vi "Characterise_Wind_Turbine.vi"(3 "Mode":T5, 5 "Traverse line In":T2 {"Row Duration (mins)" format="%#.1f"; "Row No" min=0; "Trace Gas Concentration (%)" min=0.0 format="%#.2f"; "Emission Rate (l/min)" format="%#.2f"; "Tunnel Speed" format="%#.2f"; "Start X" format="%#.2f"; "Start Y" format="%#.2f"; "Start Z" format="%#.2f"; "End X" format="%#.2f"; "End Y" format="%#.2f"; "End Z" format="%#.2f"; "Averaging time (min)" min=0.0 format="%#.2f"}) -> (0 "Error Message":string, 1 "Status":T1, 2 "Traverse line Out":T2 {"Row Duration (mins)" format="%#.1f"; "Row No" min=0; "Trace Gas Concentration (%)" min=0.0 format="%#.2f"; "Emission Rate (l/min)" format="%#.2f"; "Tunnel Speed" format="%#.2f"; "Start X" format="%#.2f"; "Start Y" format="%#.2f"; "Start Z" format="%#.2f"; "End X" format="%#.2f"; "End Y" format="%#.2f"; "End Z" format="%#.2f"; "Averaging time (min)" min=0.0 format="%#.2f"})   [LabVIEW 2010]
uses:
  Gen Trav/Multi_Run_Status.ctl
  Controls/Setup.ctl
  Controls/Save_Data.ctl
  Controls/Multi_run_mode.ctl
  Globals/Dynamic_call_global.ph.vi
  Plug in sub vis/Wind_Turbine_Global.vi
  Gen Trav/Spacing.ctl
  Gen Trav/Traverse_cluster.ctl
  Controls/User_Specific_mode.ctl
panel:
  out "Pitch Angle":dbl[](array[numeric])
  out "Array":dbl[][](array[numeric])=[[-2.5881, -0.8281, -0.8562, 5.2815, 2.845, -1.379, 0.12021, 0.04326, 0.05193, 200.0], [-3.9833, -4.1835, -3.2343, 3.6306, 1.4693, -1.9578, 0.016658, 0.014167, 0.012653, 150.0], [-9.3308, -8.7557, -8.688, 1.5839, 0.006762, -2.6254, 0.0025976, 0.0022319, 0.0025067, 100.0], [-22.4841, -21.7472, -21.4345, -1.4303, -2.2285, -3.8983, 0.00052601, 0.0020817, 0.00057503, 50.0], [-3.3014, -1.5466, -2.0325, 3.0316, -0.5057, -4.4498, 0.012392, 0.015677, 0.010797, 199.9955999515989], [-1.9125, -0.6788, -1.0112, 1.3489, -2.6429, -6.5215, 0.06848, 0.03886, 0.06433, 200.0]]
  out "Y=-200 X":dbl[](array[numeric])
  out "Y=200 X":dbl[](array[numeric])
  out "X below Highest point":dbl[](array[numeric])
  out "Yaw Angles":dbl[](array[numeric])
  out "Blade Angle":cluster{dbl[], dbl[]}[](graph)
  out "Index No":i32
  out "Current Case":string
  # "0 Blade 1 Angle\n1 Blade 2 Angle\n2 Blade 3 Angle\n3 Blade 1 Av X\n4 Blade 2 Av X\n5 Blade 3 Av X\n6 Blade 1 Var X\n7 Blade 2 Var X\n8 Blade 3 Var X\n9 Radius"
  # "X           Y            Z"
  # "Start"
  # "End"
  # "X           Y            Z"
  # "Start"
  # "End"
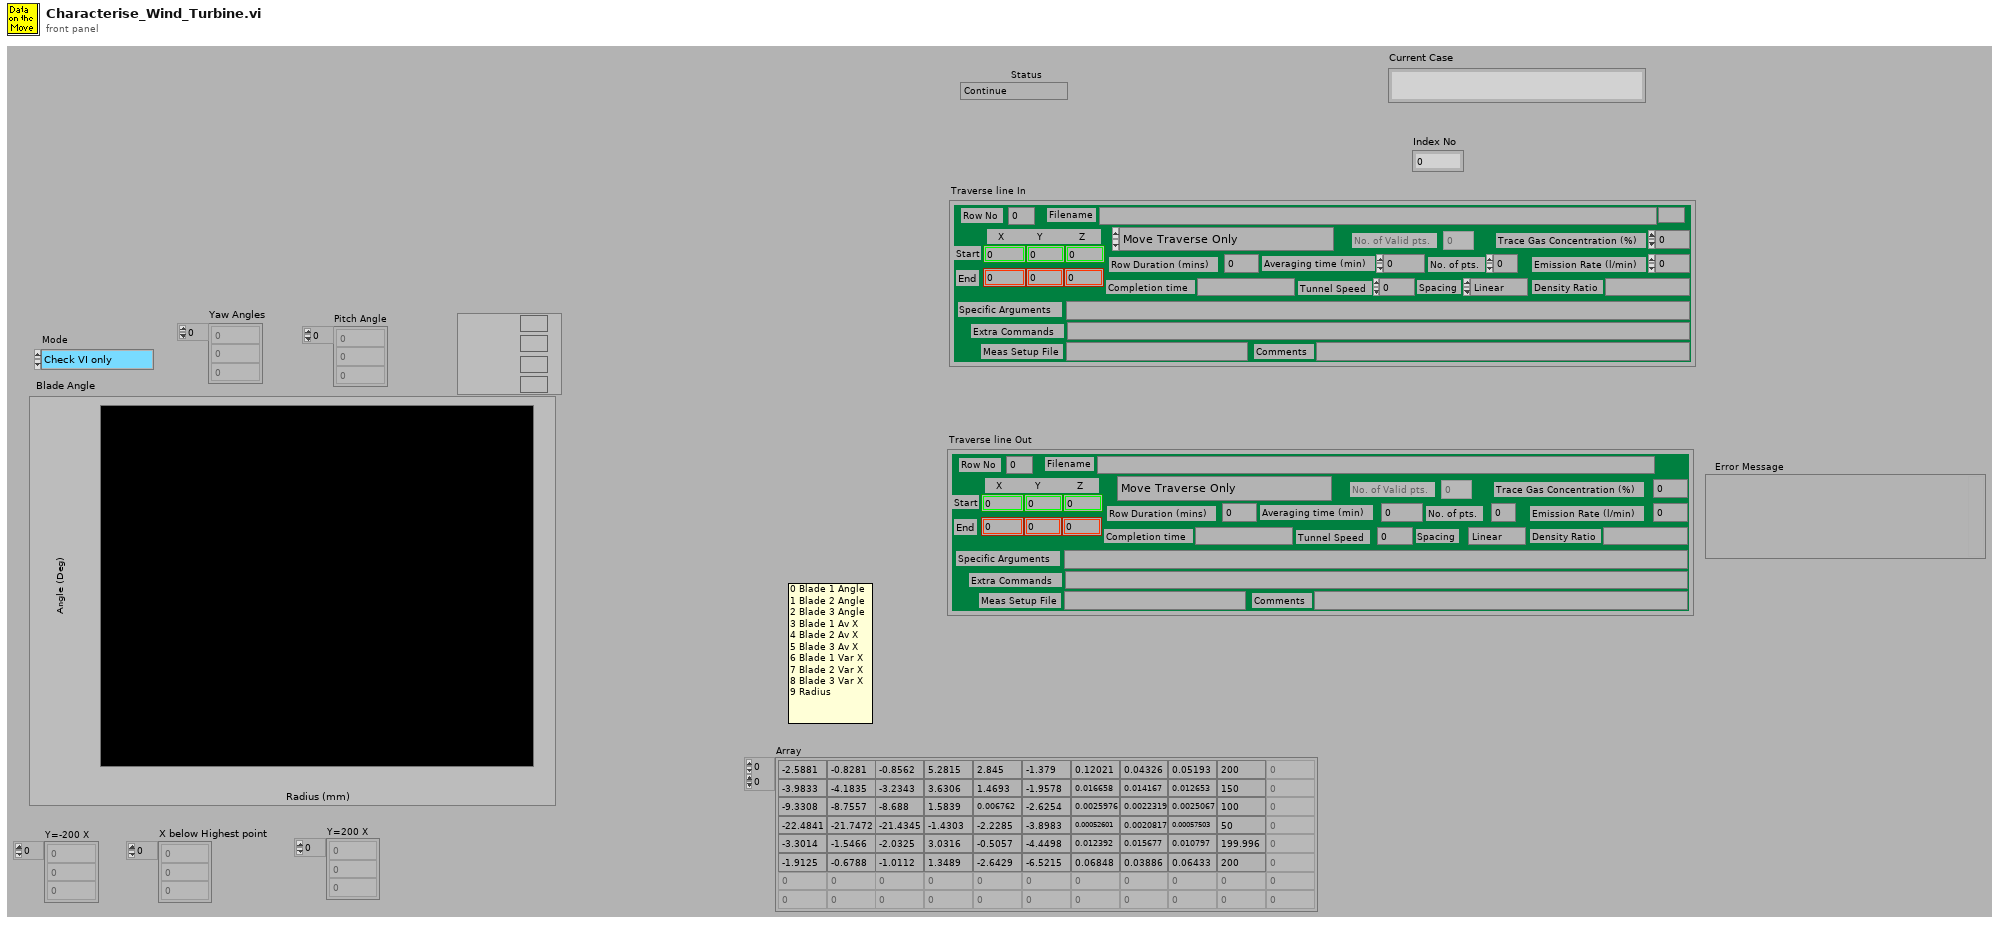
[diagram p1: front panel]
types:
  T1 = typedef "Multi_Run_Status.ctl" = enum16{"Continue", "Jump to Next Point", "Jump to Next Row", "Jump To Fall Back", "Terminate Run"}
  T2 = typedef "Traverse_cluster.ctl" = cluster{"Start X":dbl, "Start Y":dbl, "Start Z":dbl, "End X":dbl, "End Y":dbl, "End Z":dbl, "No. of pts.":i32, "Spacing":T3, "Filename":path, "Tunnel Speed":dbl, "Averaging time (min)":dbl, "Extra Commands":string, "Specific Arguments":string, "Emission Rate (l/min)":dbl, "Trace Gas Concentration (%)":dbl, "Density Ratio":string, "Comments":string, "Row No":i32, "Row Type Selector":T4, "Completion time":string, "Row Duration (mins)":dbl, "No. of Valid pts.":i32, "Meas Setup File":string}
  T3 = typedef "Spacing.ctl" = enum16{"Linear", "Log", "Gauss", "Specified", "N/A"}
  T4 = typedef "Multi_run_mode.ctl" = enum16{"Move Traverse Only", "Set Tunnel Speed Only", "Set Source Only", "Set Measurement Conditions", "Single Measurement", "Vertical Profile", "Lateral Profile", "Longitudinal Profile", "Explore Volume", "Multi-Axis Profile", "Auto Calibrate", "Meas Fast FID Bkgnd", "Check Beam Power", "Scanning Valve Measurement", "Run VI Named:", "Set ADAM Ch", "Wait (minutes)", "Send Message", "Synchronize With:", "Fall Back to this Row", "Turn Off Row Repeating", "Blank Row"}
  T5 = typedef "User_Specific_mode.ctl" = enum16{"Check VI only", "Run VI"}
  T6 = typedef "Save_Data.ctl" = enum16{"Save No Data", "Save Data"}
  T7 = typedef "Setup.ctl" = enum16{"Run Program", "Show Setup", "Save Current Setup", "Setup Front Panel"}
  T8 = typedef "Status_Cluster.ctl" = cluster{"Status":T1, "Error Type":string, "Error Description":string}
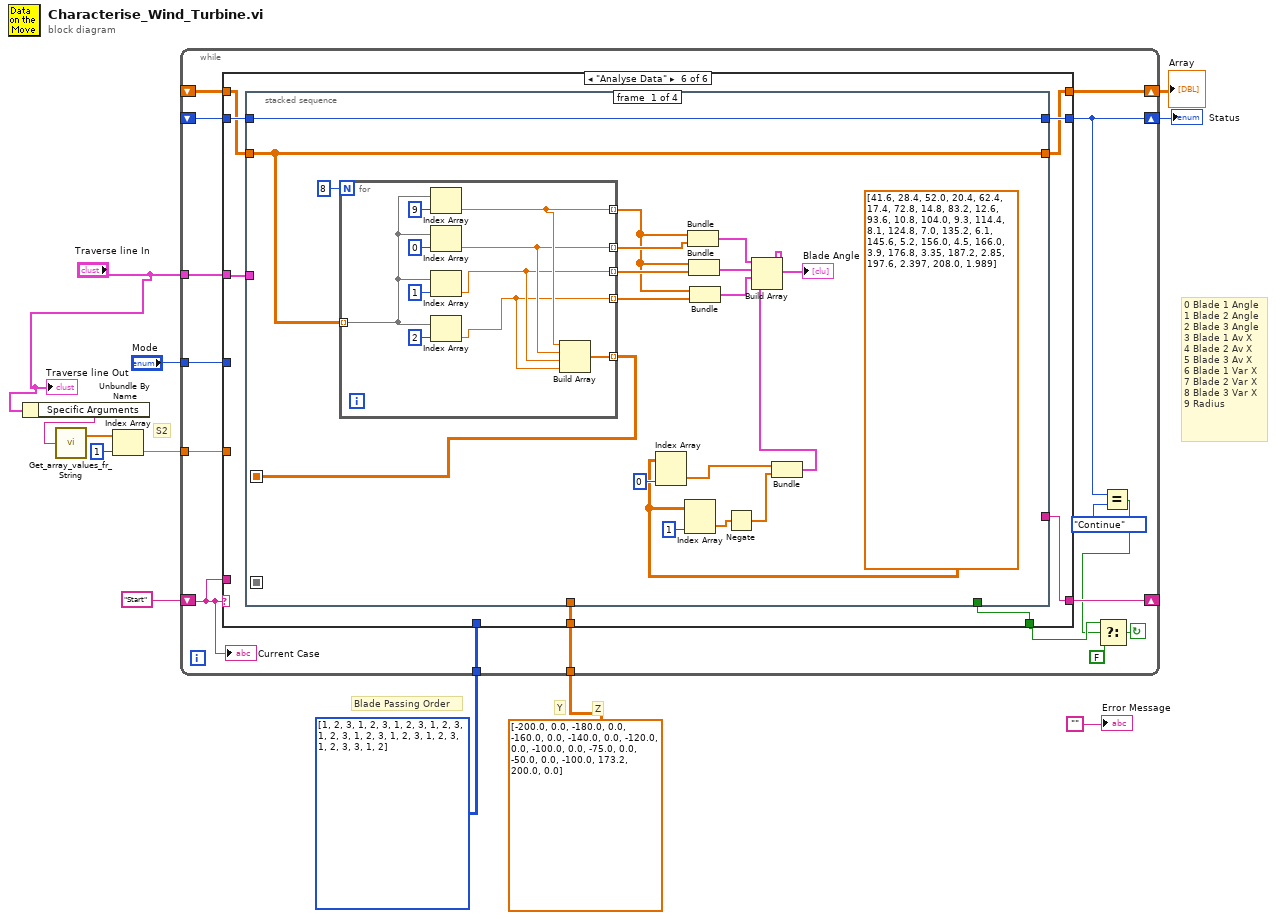
[diagram p0: block diagram]
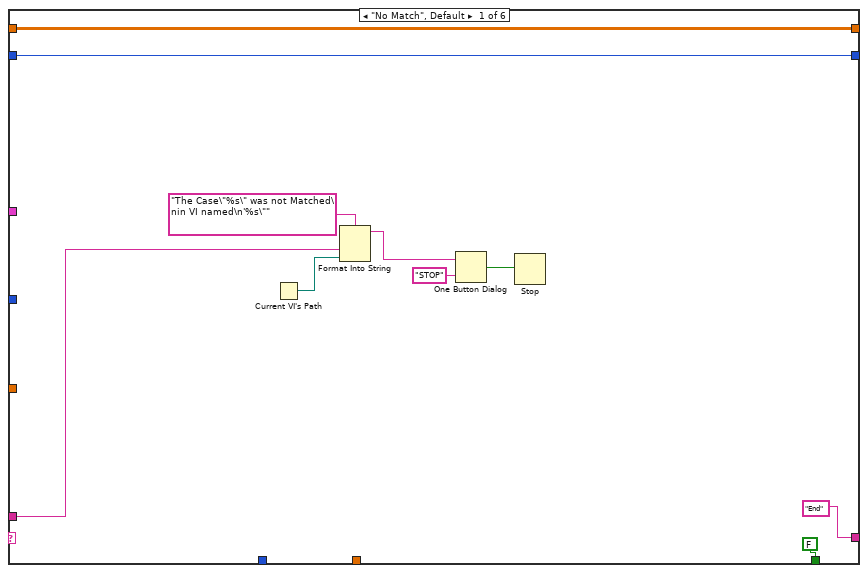
[diagram p2: hidden frame]
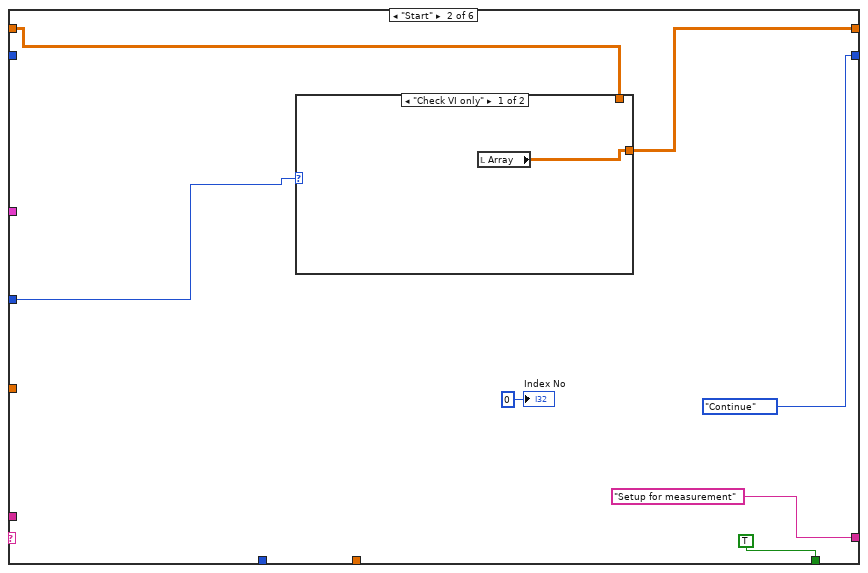
[diagram p3: hidden frame]
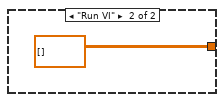
[diagram p4: hidden frame]
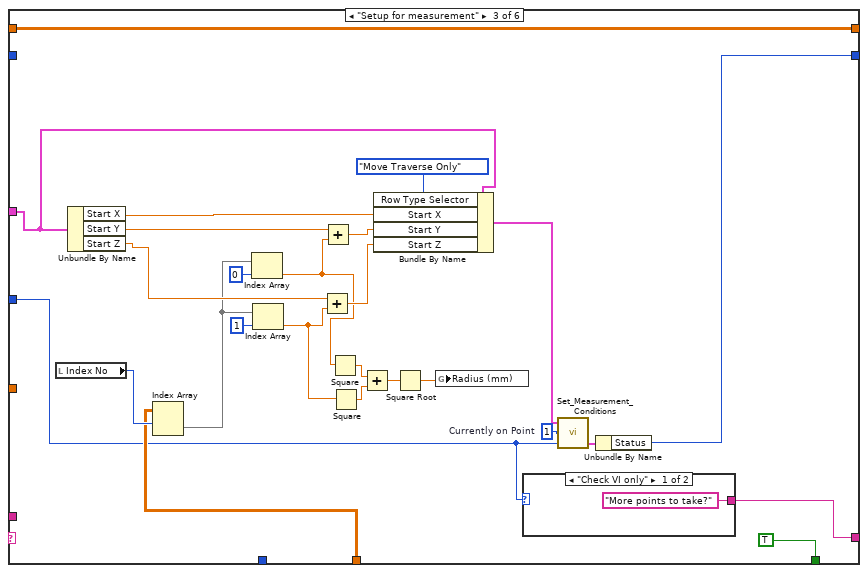
[diagram p5: hidden frame]
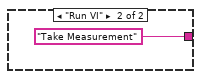
[diagram p6: hidden frame]
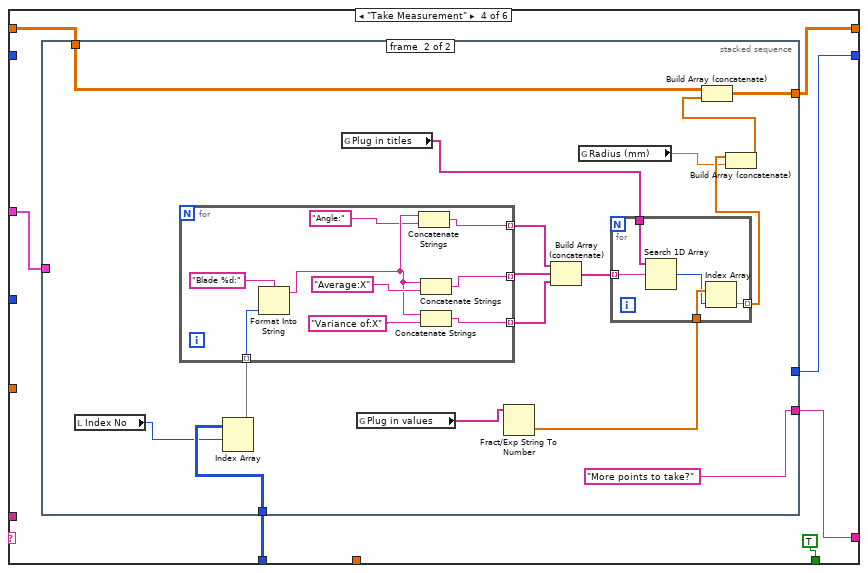
[diagram p7: hidden frame]
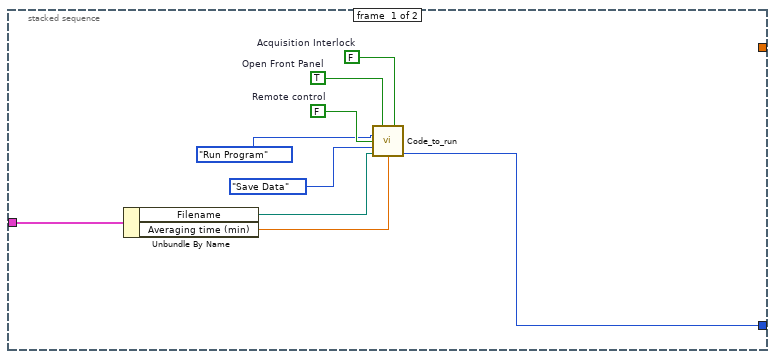
[diagram p8: hidden frame]
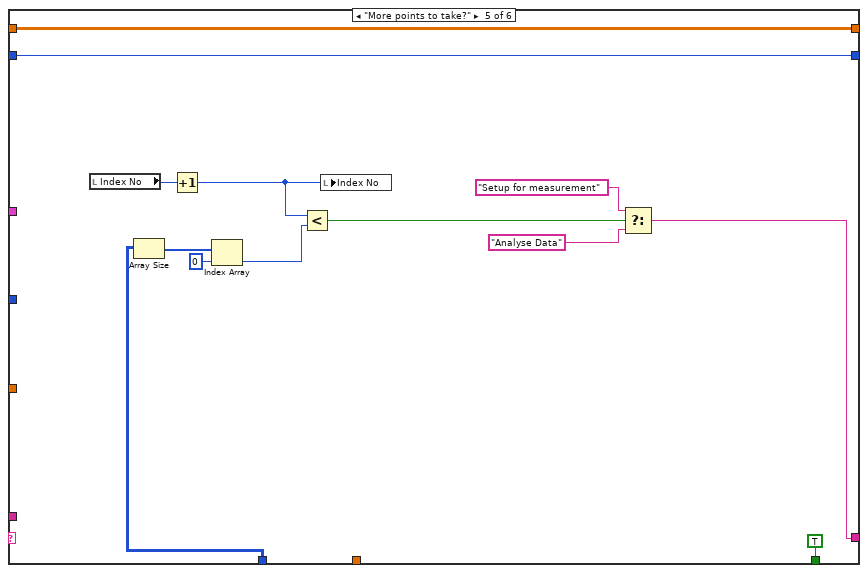
[diagram p9: hidden frame]
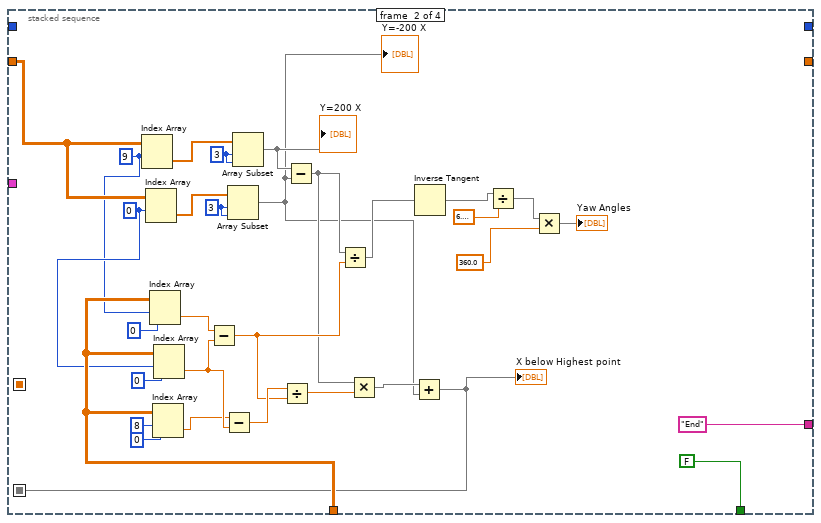
[diagram p10: hidden frame]
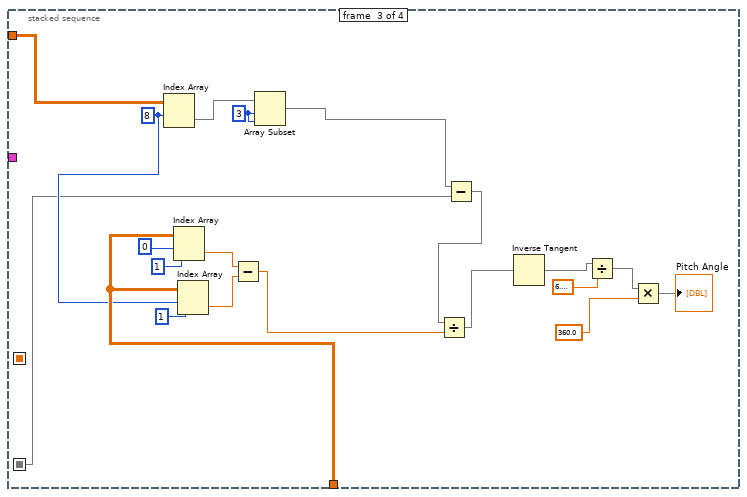
[diagram p11: hidden frame]
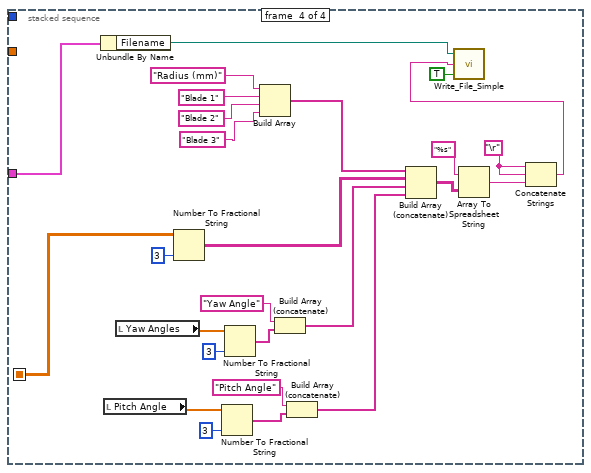
[diagram p12: hidden frame]
diagram:
  # "0 Blade 1 Angle\n1 Blade 2 Angle\n2 Blade 3 Angle\n3 Blade 1 Av X\n4 Blade 2 Av X\n5 Blade 3 Av X\n6 Blade 1 Var X\n7 Blade 2 Var X\n8 Blade 3 Var X\n9 Radius"
  # "Blade Passing Order"
  # "Z"
  # "Y"
  # "S2"
  n1 = Unbundle By Name("Traverse line In") -> ("Specific Arguments"=w5:string)
  n2 = call "Get_array_values_fr_String.vi"("String Value"=w5) -> ("Numeric Array"=w7:dbl[])  [unwired: 1 out]
  n3 = Index Array(array=w7, index=1) -> (element=w4:dbl)
  n4 = while {
    shift-left: _ -> [w26]
    shift-right: [w21] -> w10
    tunnel: "Traverse line In" -> [w27]
    tunnel: "Mode" -> [w28]
    shift-left: "Start" -> [w17]
    shift-right: [w25] -> _
    tunnel: w4 -> [w18]
    tunnel: i32[][] [[1, 2, 3], [1, 2, 3], [1, 2, 3], [1, 2, 3], [1, 2, 3], [1, 2, 3], [1, 2, 3], [1, 2, 3], [1, 2, 3], [3, 1, 2]] -> [w16]
    tunnel: dbl[][] [[-200.0, 0.0], [-180.0, 0.0], [-160.0, 0.0], [-140.0, 0.0], [-120.0, 0.0], [-100.0, 0.0], [-75.0, 0.0], [-50.0, 0.0], [-100.0, 173.2], [200.0, 0.0]] -> [w15]
    shift-right: [w14] -> w1
    shift-left: _ -> [w13]
    stop <- w19 continue-if-true
    n5 = case shown="\"Analyse Data\"" w17 {
      tunnel: w27 -> [_ _ w58 w82 _ w135]
      tunnel: w28 -> [_ w40 w48 _ _ _]
      tunnel: [FALSE ("Update Datum Powers?") TRUE ("Update Datum Powers?") TRUE ("Update Datum Powers?") TRUE ("Update Datum Powers?") TRUE ("Update Datum Powers?") w137] -> w24
      tunnel: ["End" "Setup for measurement" w70 w76 w123 w136] -> w25
      tunnel: w17 -> [w31 _ _ _ _ _]
      tunnel: w26 -> [w30 _ _ _ w125 w141]
      tunnel: [w30 Multi_Run_Status."Continue" ("Status") w71 w80 w125 w142] -> w21
      tunnel: w18 -> [_ _ _ _ _ _]
      tunnel: w16 -> [_ _ _ w79 w124 _]
      tunnel: w15 -> [_ _ w60 _ _ w138]
      tunnel: [w29 w41 w50 w78 w126 w140] -> w14
      tunnel: w13 -> [w29 w39 w50 w77 w126 w139]
      frame "No Match", Default {
        n6 = Current VI's Path() -> (path=w34:path)
        n7 = Format Into String(format string="The Case\"%s\" was not Matched\nin VI named\n'%s\"" ("Format String"), w31, w34) -> (resulting string=w37:string)  [unwired: 2 in, 1 out]
        n8 = One Button Dialog(message=w37, button name ("OK")="STOP") -> (true=w35:bool)
        n9 = Stop(stop? (T)=w35) -> ()
      }
      frame "Start" {
        n10 = case shown="\"Check VI only\"" w40 {
          tunnel: [w46 dbl[][] []] -> w41
          tunnel: w39 -> [_ _]
          frame "Check VI only" {
            n11 = local read "Array"() -> (w46:dbl[][])
          }
          frame "Run VI" {
          }
        }
        "Index No" <- 0 ("Index No")
      }
      frame "Setup for measurement" {
        w72 = 1  # Currently on Point
        n12 = local read "Index No"() -> (w61:i32)
        n13 = Unbundle By Name(w58) -> ("Start X"=w69:dbl, "Start Y"=w67:dbl, "Start Z"=w68:dbl)
        n14 = Index Array(array=w60, index (row)=w61) -> (element=w59:dbl[])  [unwired: 1 in]
        n15 = Index Array(array=w59, index=0) -> (element=w56:dbl)
        n16 = Index Array(array=w59, index=1) -> (element=w55:dbl)
        n17 = Add(x=w68, y=w55) -> (x+y=w62:dbl)
        n18 = Add(x=w67, y=w56) -> (x+y=w63:dbl)
        n19 = Square(x=w56) -> (x^2=w54:dbl)
        n20 = Square(x=w55) -> (x^2=w53:dbl)
        n21 = Add(x=w54, y=w53) -> (x+y=w52:dbl)
        n22 = Bundle By Name(cluster=w58, "Row Type Selector"=Multi_run_mode."Move Traverse Only", "Start X"=w69, "Start Y"=w63, "Start Z"=w62) -> (w57:T2)
        n23 = Square Root(x=w52) -> (sqrt(x)=w51:dbl)
        n24 = global write "Wind_Turbine_Global.vi" "Radius (mm)"(w51) -> ()
        n25 = case shown="\"Check VI only\"" w48 {
          tunnel: ["More points to take?" "Take Measurement"] -> w70
          frame "Check VI only" {
          }
          frame "Run VI" {
          }
        }
        n26 = call "Set_Measurement_Conditions.vi"("Simulate/Run"=w48, "Currently on Point"=w72, "Traverse line"=w57) -> ("Status Cluster"=w73:T8)  [unwired: 2 out]
        n27 = Unbundle By Name(w73) -> ("Status"=w71:T1)
      }
      frame "Take Measurement" {
        n28 = stacked-sequence {
          tunnel: [w91 _] -> w80
          tunnel: w82 -> [w90 _]
          tunnel: w79 -> [_ w107]
          tunnel: [_ w99] -> w78
          tunnel: w77 -> [_ w98]
          tunnel: [_ "More points to take?"] -> w76
          frame #0 {
            w86 = FALSE  # Acquisition Interlock
            w87 = TRUE  # Open Front Panel
            w89 = FALSE  # Remote control
            n29 = Unbundle By Name(w90) -> ("Filename"=w83:path, "Averaging time (min)"=w88:dbl)
            n30 = call "Code_to_run.vi"("Open Front Panel"=w87, "Acquisition Interlock"=w86, "setup"=Setup."Run Program", "Remote control"=w89, "File"=Save_Data."Save Data", "Results Filename"=w83, "Averaging time (min)"=w88) -> ("Status"=w91:T1)  [unwired: 4 in, 4 out]
          }
          frame #1 {
            n31 = local read "Index No"() -> (w106:i32)
            n32 = Index Array(array=w107, index (row)=w106) -> (element=w105:i32[])  [unwired: 1 in]
            n33 = for {
              tunnel: [w118] -> w103 mode=indexing
              tunnel: [w117] -> w102 mode=indexing
              tunnel: [w116] -> w104 mode=indexing
              tunnel: w105 -> [w113] mode=indexing
              n34 = Format Into String(format string="Blade %d:", w113) -> (resulting string=w115:string)  [unwired: 2 in, 1 out]
              n35 = Concatenate Strings(w115, "Angle:") -> (w116:string)
              n36 = Concatenate Strings(w115, "Average:X") -> (w118:string)
              n37 = Concatenate Strings(w115, "Variance of:X") -> (w117:string)
            }
            n38 = global read "Dynamic_call_global.ph.vi" "Plug in titles"() -> (w101:string[])
            n39 = global read "Dynamic_call_global.ph.vi" "Plug in values"() -> (w97:string[])
            n40 = Fract/Exp String To Number(string=w97) -> (number=w96:dbl[])  [unwired: 3 in, 1 out]
            n41 = Build Array (concatenate)(w104, w103, w102) -> (w100:string[])
            n42 = global read "Wind_Turbine_Global.vi" "Radius (mm)"() -> (w94:dbl)
            n43 = for {
              tunnel: w101 -> [w112]
              tunnel: w100 -> [w111] mode=indexing
              tunnel: w96 -> [w110]
              tunnel: [w108] -> w95 mode=indexing
              n44 = Search 1D Array(1D array=w112, element=w111) -> (index of element=w109:i32)  [unwired: 1 in]
              n45 = Index Array(array=w110, index=w109) -> (element=w108:dbl)
            }
            n46 = Build Array (concatenate)(w95, w94) -> (w93:dbl[])
            n47 = Build Array (concatenate)(w98, w93) -> (w99:dbl[][])
          }
        }
      }
      frame "More points to take?" {
        n48 = local read "Index No"() -> (w132:i32)
        n49 = Array Size(array=w124) -> (size(s)=w134:i32[])
        n50 = Increment(x=w132) -> (x+1=w131:i32)
        n51 = Index Array(array=w134, index=0) -> (element=w130:i32)
        n52 = Less?(x=w131, y=w130) -> (x < y?=w129:bool)
        n53 = local write "Index No"(w131) -> ()
        n54 = Select(t="Setup for measurement", s=w129, f="Analyse Data") -> (s? t:f=w123:string)
      }
      frame "Analyse Data" {
        n55 = stacked-sequence {
          seq-local: [_ w172 _ _] -> [_ _ w211 _]
          seq-local: [w145 _ _ _] -> [_ _ _ w245]
          tunnel: [w161 _ _ _] -> w142
          tunnel: w141 -> [w161 _ _ _]
          tunnel: [w159 _ _ _] -> w140
          tunnel: w139 -> [w159 w202 w220 _]
          tunnel: w138 -> [_ w188 w215 _]
          tunnel: [_ FALSE _ _] -> w137
          tunnel: [_ "End" _ _] -> w136
          tunnel: w135 -> [_ _ _ w247]
          frame #0 {
            w151 = dbl[][] [[41.6, 28.4], [52.0, 20.4], [62.4, 17.4], [72.8, 14.8], [83.2, 12.6], [93.6, 10.8], [104.0, 9.3], [114.4, 8.1], [124.8, 7.0], [135.2, 6.1], [145.6, 5.2], [156.0, 4.5], [166.0, 3.9], [176.8, 3.35], [187.2, 2.85], [197.6, 2.397], [208.0, 1.989]]
            n56 = for {
              N: 8 -> [_]
              tunnel: w159 -> [w167] mode=indexing
              tunnel: [w166] -> w146 mode=indexing
              tunnel: [w165] -> w149 mode=indexing
              tunnel: [w164] -> w147 mode=indexing
              tunnel: [w163] -> w148 mode=indexing
              tunnel: [w162] -> w145 mode=indexing
              n57 = Index Array(array=w167, index=9) -> (element=w166:dbl)
              n58 = Index Array(array=w167, index=0) -> (element=w165:dbl)
              n59 = Index Array(array=w167, index=1) -> (element=w164:dbl)
              n60 = Index Array(array=w167, index=2) -> (element=w163:dbl)
              n61 = Build Array(w166, w165, w164, w163) -> (w162:dbl[])
            }
            n62 = Index Array(array=w151, index (col)=0 ("disabled index (col)")) -> (element=w153:dbl[])  [unwired: 1 in]
            n63 = Index Array(array=w151, index (col)=1 ("disabled index (col)")) -> (element=w144:dbl[])  [unwired: 1 in]
            n64 = Bundle(w146, w149) -> (w158:cluster{dbl[], dbl[]})  [unwired: 1 in]
            n65 = Bundle(w146, w147) -> (w157:cluster{dbl[], dbl[]})  [unwired: 1 in]
            n66 = Bundle(w146, w148) -> (w156:cluster{dbl[], dbl[]})  [unwired: 1 in]
            n67 = Negate(x=w144) -> (-x=w143:dbl[])
            n68 = Bundle(w153, w143) -> (w150:cluster{dbl[], dbl[]})  [unwired: 1 in]
            n69 = Build Array(w158, w157, w156, w150) -> (→"Blade Angle":cluster{dbl[], dbl[]}[])
          }
          frame #1 {
            w199 = 3 ("index")
            w201 = 3 ("index")
            w184 = 0 ("index (row)")
            w183 = 9 ("index (row)")
            n70 = Index Array(array=w202, index (row)=w183) -> (element=w200:dbl[])  [unwired: 1 in]
            n71 = Index Array(array=w202, index (row)=w184) -> (element=w179:dbl[])  [unwired: 1 in]
            n72 = Index Array(array=w188, index (row)=w183, index (col)=0 ("disabled index (col)")) -> (element=w187:dbl)
            n73 = Index Array(array=w188, index (row)=8, index (col)=0 ("disabled index (col)")) -> (element=w175:dbl)
            n74 = Index Array(array=w188, index (row)=w184, index (col)=0 ("disabled index (col)")) -> (element=w176:dbl)
            n75 = Subtract(x=w187, y=w176) -> (x-y=w185:dbl)
            n76 = Subtract(x=w175, y=w176) -> (x-y=w186:dbl)
            n77 = Array Subset(array=w179, index=w199, length=w199) -> (w173:dbl[])
            "Y=-200 X" <- w173
            n78 = Array Subset(array=w200, index=w201, length=w201) -> (w174:dbl[])
            "Y=200 X" <- w174
            n79 = Divide(x=w186, y=w185) -> (x/y=w181:dbl)
            n80 = Subtract(x=w174, y=w173) -> (x-y=w182:dbl[])
            n81 = Divide(x=w182, y=w185) -> (x/y=w194:dbl[])
            n82 = Multiply(x=w182, y=w181) -> (x*y=w180:dbl[])
            n83 = Add(x=w180, y=w173) -> (x+y=w172:dbl[])
            "X below Highest point" <- w172
            n84 = Inverse Tangent(1:w194) -> (0:w195:dbl[])
            n85 = Divide(x=w195, y=6.283185307179586) -> (x/y=w192:dbl[])
            n86 = Multiply(x=w192, y=360.0) -> (x*y=→"Yaw Angles":dbl[])
          }
          frame #2 {
            w222 = 3 ("index")
            w213 = 8 ("index (row)")
            n87 = Index Array(array=w220, index (row)=w213) -> (element=w221:dbl[])  [unwired: 1 in]
            n88 = Index Array(array=w215, index (row)=0 ("disabled index (col)"), index (col)=1 ("disabled index (col)")) -> (element=w217:dbl)
            n89 = Index Array(array=w215, index (row)=w213, index (col)=1 ("disabled index (col)")) -> (element=w216:dbl)
            n90 = Subtract(x=w217, y=w216) -> (x-y=w205:dbl)
            n91 = Array Subset(array=w221, index=w222, length=w222) -> (w212:dbl[])
            n92 = Subtract(x=w212, y=w211) -> (x-y=w204:dbl[])
            n93 = Divide(x=w204, y=w205) -> (x/y=w208:dbl[])
            n94 = Inverse Tangent(1:w208) -> (0:w209:dbl[])
            n95 = Divide(x=w209, y=6.283185307179586) -> (x/y=w206:dbl[])
            n96 = Multiply(x=w206, y=360.0) -> (x*y=→"Pitch Angle":dbl[])
          }
          frame #3 {
            w225 = "\r"
            n97 = Unbundle By Name(w247) -> ("Filename"=w246:path)
            n98 = local read "Pitch Angle"() -> (w234:dbl[])
            n99 = local read "Yaw Angles"() -> (w236:dbl[])
            n100 = Number To Fractional String(number=w245, precision (6)=i16 3) -> (F-format string=w238:string[][])  [unwired: 2 in]
            n101 = Number To Fractional String(number=w234, precision (6)=i16 3) -> (F-format string=w231:string[])  [unwired: 2 in]
            n102 = Number To Fractional String(number=w236, precision (6)=i16 3) -> (F-format string=w233:string[])  [unwired: 2 in]
            n103 = Build Array("Radius (mm)", "Blade 1", "Blade 2", "Blade 3") -> (w239:string[])
            n104 = Build Array (concatenate)("Yaw Angle", w233) -> (w229:string[])
            n105 = Build Array (concatenate)("Pitch Angle", w231) -> (w228:string[])
            n106 = Build Array (concatenate)(w239, w238, w229, w228) -> (w227:string[][])
            n107 = Array To Spreadsheet String(array=w227, 3:"%s" ("format string")) -> (spreadsheet string=w226:string)  [unwired: 1 in]
            n108 = Concatenate Strings(w225, w225, w226) -> (w224:string)
            n109 = call "Write_File_Simple.vi"("append to file? (new file:F)"=TRUE, "character string"=w224, "file path"=w246) -> ()  [unwired: 2 out]
          }
        }
      }
    }
    n110 = Equal?(x=w21, y=Multi_Run_Status."Continue" ("Status")) -> (x = y?=w23:bool)
    n111 = Select(t=w24, s=w23, f=FALSE) -> (s? t:f=w19:bool)
    "Current Case" <- w17
  }
  "Status" <- w10
  "Array" <- w1
  "Error Message" <- ""
  "Traverse line Out" <- "Traverse line In"
